vi "INIT.vi"(8 "error in (no error)":errorcluster, 11 "Detector in":refnum<class "Detector.lvclass">) -> (0 "error out":errorcluster, 3 "Detector out":refnum<class "Detector.lvclass">)   [LabVIEW 2019, in "Detector.lvclass"]
uses:
  Detector.lvclass
  C:/Users/elysium/Documents/dev/TRANCON/Classes/GeneralFunctionality/GeneralFunctionality.lvclass
  GeneralFunctionality/GeneralFunctionality.lvclass/GeneralFunctionality.ctl
  GeneralFunctionality/GeneralFunctionality.lvclass
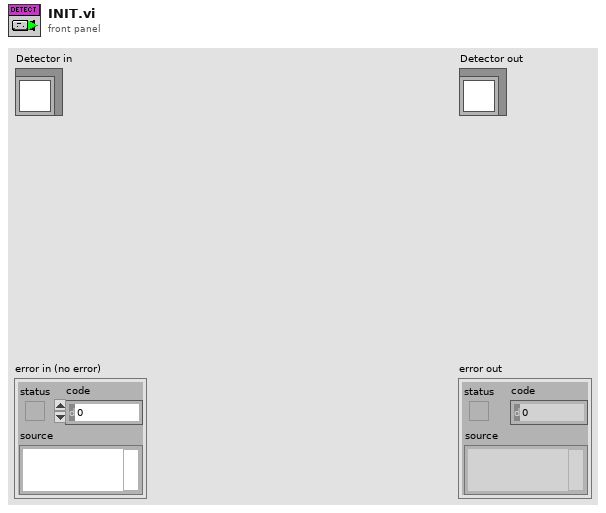
[diagram p1: front panel]
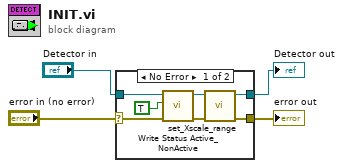
[diagram p0: block diagram]
diagram:
  n1 = case shown="No Error" "error in (no error)" {
    selector: "error in (no error)" -> [w9 w12]
    tunnel: "Detector in" -> [w10 w13]
    tunnel: [w5 w13] -> w2
    tunnel: [w6 w12] -> w1
    frame No Error {
      n2 = call "Write Status Active_NonActive.vi"("error in (no error)"=w9, "Status Active/NonActive"=TRUE, "GeneralFunctionality in"=w10) -> ("error out"=w8:errorcluster, "GeneralFunctionality out"=w7:refnum<class "Detector.lvclass">)  [unwired: 7 in]
      n3 = call "set_Xscale_range.vi"("error in (no error)"=w8, "Detector in"=w7) -> ("error out"=w6:errorcluster, "Detector out"=w5:refnum<class "Detector.lvclass">)  [unwired: 8 in]
    }
    frame Error {
    }
  }
  "error out" <- w1
  "Detector out" <- w2
